vi "svc_Extract Numerator and Denominator Unit Labels.vi"(0 "unit label":string="(in/s^2)/(m/s^2)") -> (4 "numerator unit label":string, 6 "denominator unit label":string)   [LabVIEW 2017]
doc: "This VI extracts <B>numerator unit label</B> and <B>denominator unit label</B> from the linear portion of the <B>unit label</B> contained in the spectrum info."
panel:
  out "den 2":string
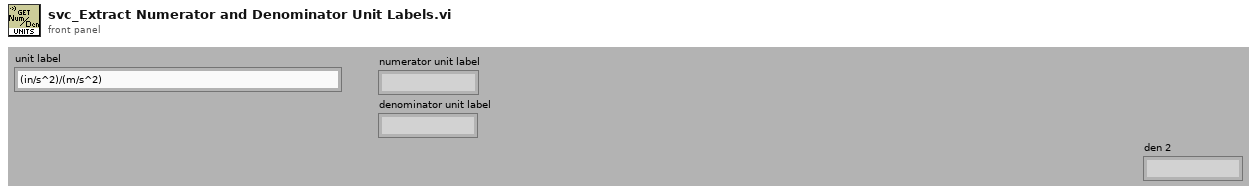
[diagram p1: front panel]
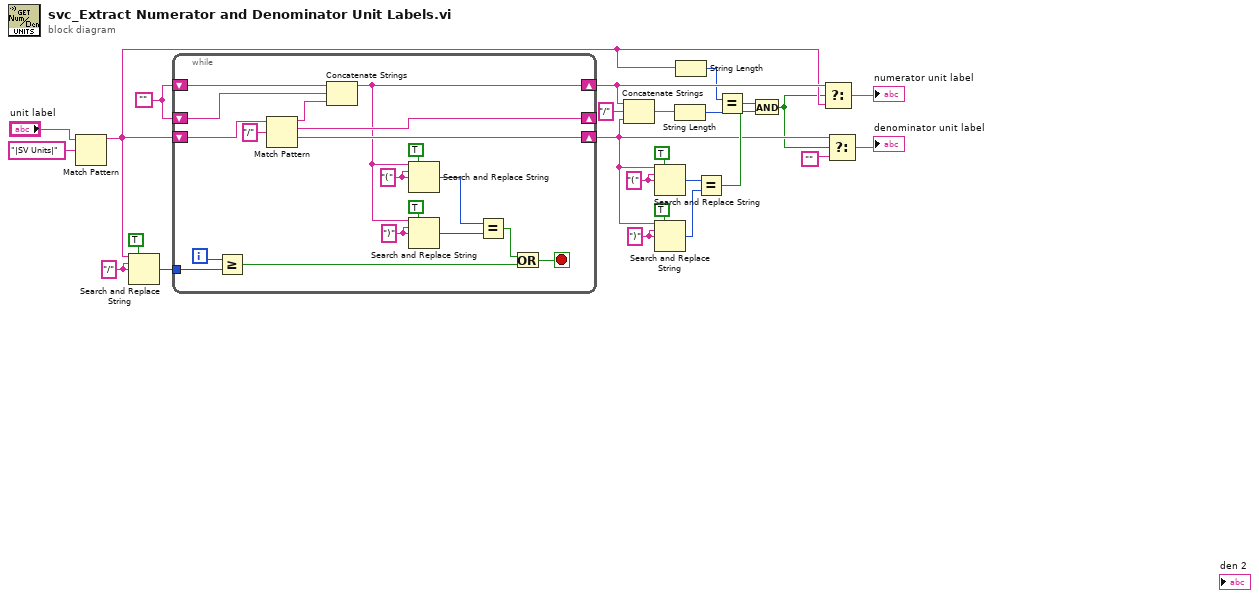
[diagram p0: block diagram]
diagram:
  w16 = ")" ("regular expression")
  w17 = "(" ("regular expression")
  w20 = ""
  w22 = "/" ("regular expression")
  n1 = Match Pattern(string="unit label", regular expression="|SV Units|" ("string")) -> (before substring=w5:string)  [unwired: 1 in, 3 out]
  n2 = Search and Replace String(replace all?=TRUE ("replace all? (F)"), input string=w5, search string=w22, replace string=w22) -> (number of replacements=w21:i32)  [unwired: 4 in, 3 out]
  n3 = while {
    tunnel: w21 -> [w43]
    shift-right: [w29] -> w8
    shift-left: w5 -> [w35]
    shift-right: [w26] -> w9
    shift-left: w20 -> [w31]
    shift-right: [w27] -> _
    shift-left: w20 -> [w30]
    i -> [w44]
    stop <- w34 stop-if-true
    w39 = ")" ("regular expression")
    w38 = "(" ("regular expression")
    n4 = Greater Or Equal?(x=w44, y=w43) -> (x >= y?=w32:bool)
    n5 = Match Pattern(string=w35, regular expression="/") -> (before substring=w28:string, match substring=w27:string, after substring=w29:string)  [unwired: 1 in, 1 out]
    n6 = Concatenate Strings(w31, w30, w28) -> (w26:string)
    n7 = Search and Replace String(replace all?=TRUE ("replace all? (F)"), input string=w26, search string=w38, replace string=w38) -> (number of replacements=w41:i32)  [unwired: 4 in, 3 out]
    n8 = Search and Replace String(replace all?=TRUE ("replace all? (F)"), input string=w26, search string=w39, replace string=w39) -> (number of replacements=w42:i32)  [unwired: 4 in, 3 out]
    n9 = Equal?(x=w41, y=w42) -> (x = y?=w33:bool)
    n10 = Or(x=w33, y=w32) -> (x .or. y?=w34:bool)
  }
  n11 = Concatenate Strings(w9, "/" ("regular expression"), w8) -> (w6:string)
  n12 = Search and Replace String(replace all?=TRUE ("replace all? (F)"), input string=w8, search string=w17, replace string=w17) -> (number of replacements=w14:i32)  [unwired: 4 in, 3 out]
  n13 = Search and Replace String(replace all?=TRUE ("replace all? (F)"), input string=w8, search string=w16, replace string=w16) -> (number of replacements=w13:i32)  [unwired: 4 in, 3 out]
  n14 = String Length(string=w6) -> (length=w4:i32)
  n15 = String Length(string=w5) -> (length=w3:i32)
  n16 = Equal?(x=w14, y=w13) -> (x = y?=w10:bool)
  n17 = Equal?(x=w3, y=w4) -> (x = y?=w2:bool)
  n18 = And(x=w2, y=w10) -> (x .and. y?=w1:bool)
  n19 = Select(t=w9, s=w1, f=w5) -> (s? t:f=→"numerator unit label":string)
  n20 = Select(t=w8, s=w1, f="") -> (s? t:f=→"denominator unit label":string)
